vi "DSF.Engine.Execution.Framework.Get Configuration.vi"(8 "error in (no error)":errorcluster, 11 "Framework in":refnum<class "DSF.Engine.Execution.Framework.lvclass">) -> (0 "error out":errorcluster, 2 "Framework Configuration":refnum<class "DSF.Shared.Configuration.Framework.lvclass">, 3 "Framework out":refnum<class "DSF.Engine.Execution.Framework.lvclass">)   [LabVIEW 2016, in "DSF.Engine.lvlib" / "DSF.Engine.Execution.Framework.lvclass"]
uses:
  DSF.Engine.Execution.Framework.lvclass
  Shared/Classes/Framework/DSF.Shared.Configuration.Framework.lvclass
  DSF.Engine.Execution.Framework.lvclass/DSF.Engine.Execution.Framework.ctl
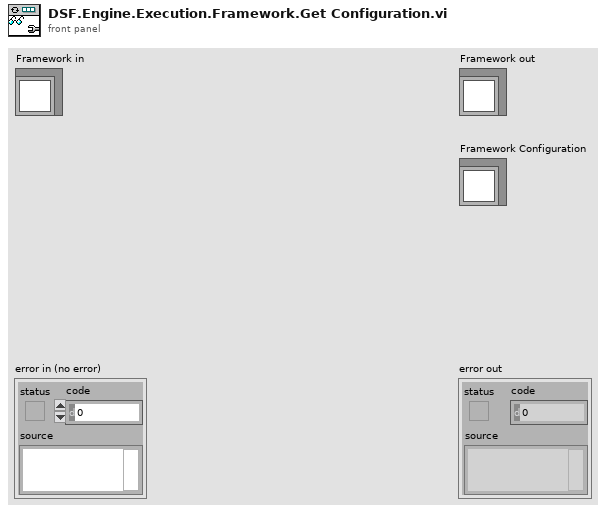
[diagram p1: front panel]
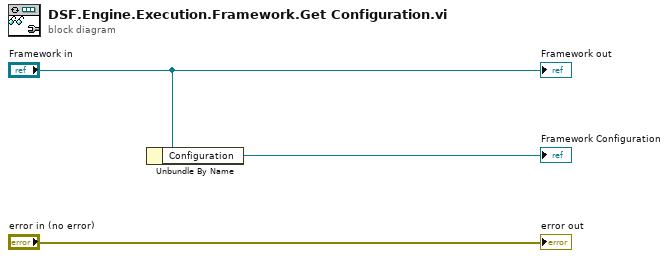
[diagram p0: block diagram]
diagram:
  n1 = Unbundle By Name("Framework in") -> ("Configuration"=→"Framework Configuration":refnum<class "DSF.Shared.Configuration.Framework.lvclass">)
  "error out" <- "error in (no error)"
  "Framework out" <- "Framework in"
